vi "Ev Reset Path.vi"(8 "error in (no error)":errorcluster, 11 "Configuration Window in":refnum<class "Configuration Window.lvclass">) -> (0 "error out":errorcluster, 3 "Configuration Window out":refnum<class "Configuration Window.lvclass">)   [LabVIEW 2018, in "Configuration Window.lvlib" / "Configuration Window.lvclass"]
uses:
  Configuration Window.lvclass
  Configuration Window.lvclass/Configuration Window.ctl
  Main Panel/LF2R IDE/LF2R IDE.lvclass
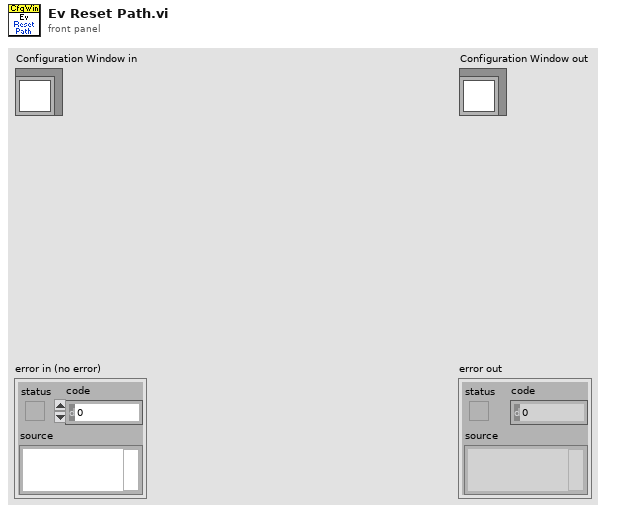
[diagram p1: front panel]
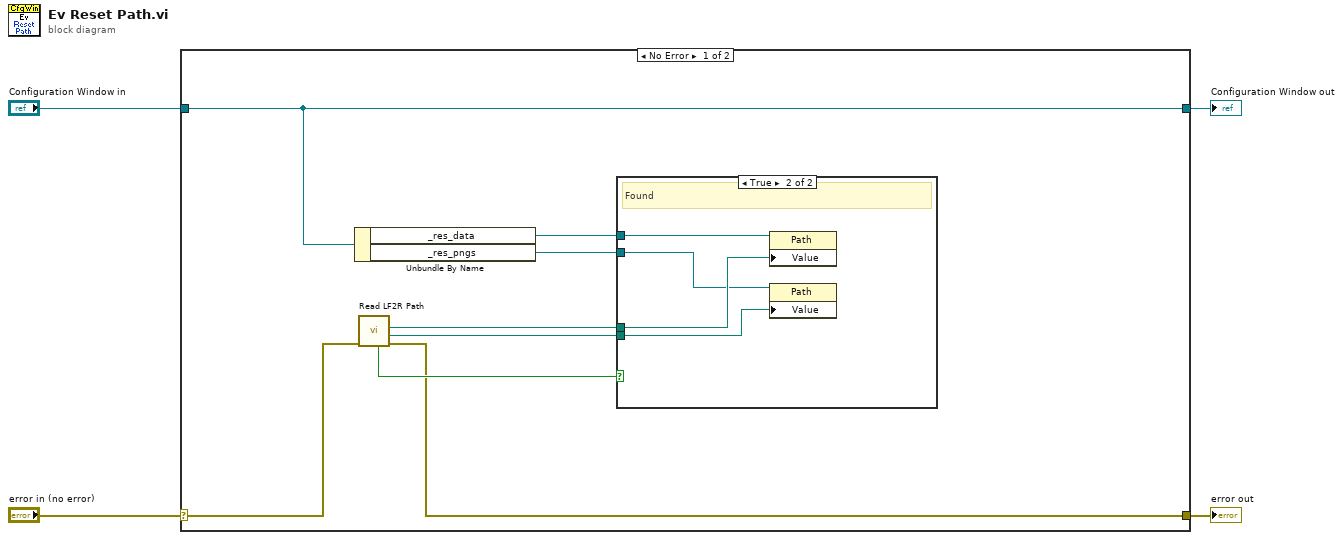
[diagram p0: block diagram]
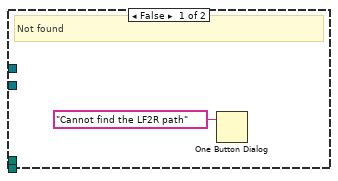
[diagram p2: hidden frame]
diagram:
  n1 = case shown="No Error" "error in (no error)" {
    selector: "error in (no error)" -> [w5 w19]
    tunnel: [w6 w19] -> w3
    tunnel: [w12 w18] -> w1
    tunnel: "Configuration Window in" -> [w12 w18]
    frame No Error {
      n2 = Unbundle By Name(w12) -> ("_res_data"=w11:refnum<vi>, "_res_pngs"=w9:refnum<vi>)
      n3 = call "Read LF2R Path.vi"("error in (no error)"=w5) -> ("error out"=w6:errorcluster, "PNG Path"=w8:path, "Data Path"=w10:path, "Found"=w7:bool)  [unwired: 6 in, 1 out]
      n4 = case shown="True" w7 {
        tunnel: w11 -> [_ w17]
        tunnel: w10 -> [_ w16]
        tunnel: w9 -> [_ w15]
        tunnel: w8 -> [_ w14]
        frame False {
          # "Not found"
          n5 = One Button Dialog(message="Cannot find the LF2R path") -> ()  [unwired: 1 in, 1 out]
        }
        frame True {
          # "Found"
          n6 = property class="Path"(reference=w17, "Value"=w16) -> ()  [unwired: 1 in, 2 out]
          n7 = property class="Path"(reference=w15, "Value"=w14) -> ()  [unwired: 1 in, 2 out]
        }
      }
    }
    frame Error {
    }
  }
  "error out" <- w3
  "Configuration Window out" <- w1
